vi "Computer.vi"() -> ()   [LabVIEW 2012]
uses:
  <vilib>/Utility/inputDevices.llb/closeJoystick.vi
  <vilib>/Utility/inputDevices.llb/joystickAcquire.vi
panel:
  out "TX Data":T1
  in  "ESTOP":bool
  in  "Robot Port":u16=2055 min=1025 step=1
  in  "Robot Address":string="192.168.1.200"
  in  "stop":bool
  # "Computer Control"
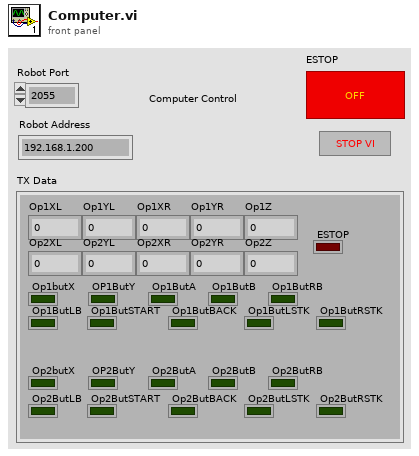
[diagram p1: front panel]
types:
  T1 = cluster{"Op2ButLSTK":bool, "Op2ButRSTK":bool, "Op1ButLSTK":bool, "Op1ButRSTK":bool, "Op1XL":i32, "Op1YL":i32, "Op1XR":i32, "Op1YR":i32, "Op1Z":i32, "Op2XL":i32, "Op2YL":i32, "Op2XR":i32, "Op2YR":i32, "Op2Z":i32, "ESTOP":bool, "Op1butX":bool, "OP1ButY":bool, "Op1ButA":bool, "Op1ButB":bool, "Op1ButRB":bool, "Op1ButLB":bool, "Op2butX":bool, "OP2ButY":bool, "Op2ButA":bool, "Op2ButB":bool, "Op2ButRB":bool, "Op2ButLB":bool, "Op2ButSTART":bool, "Op2ButBACK":bool, "Op1ButSTART":bool, "Op1ButBACK":bool}
  T2 = cluster{"X axis":i32, "Y axis":i32, "Z axis":i32, "X axis rotation":i32, "Y axis rotation":i32, "Z axis rotation":i32, "U axis":i32, "V axis":i32}
  T3 = cluster{"button 1":bool, "button 2":bool, "button 3":bool, "button 4":bool, "button 5":bool, "button 6":bool, "button 7":bool, "button 8":bool, "button 9":bool, "button 10":bool, "button 11":bool, "button 12":bool, "button 13":bool, "button 14":bool, "button 15":bool, "button 16":bool, "button 17":bool, "button 18":bool, "button 19":bool, "button 20":bool, "button 21":bool, "button 22":bool, "button 23":bool, "button 24":bool, "button 25":bool, "button 26":bool, "button 27":bool, "button 28":bool, "button 29":bool, "button 30":bool, "button 31":bool, "button 32":bool}
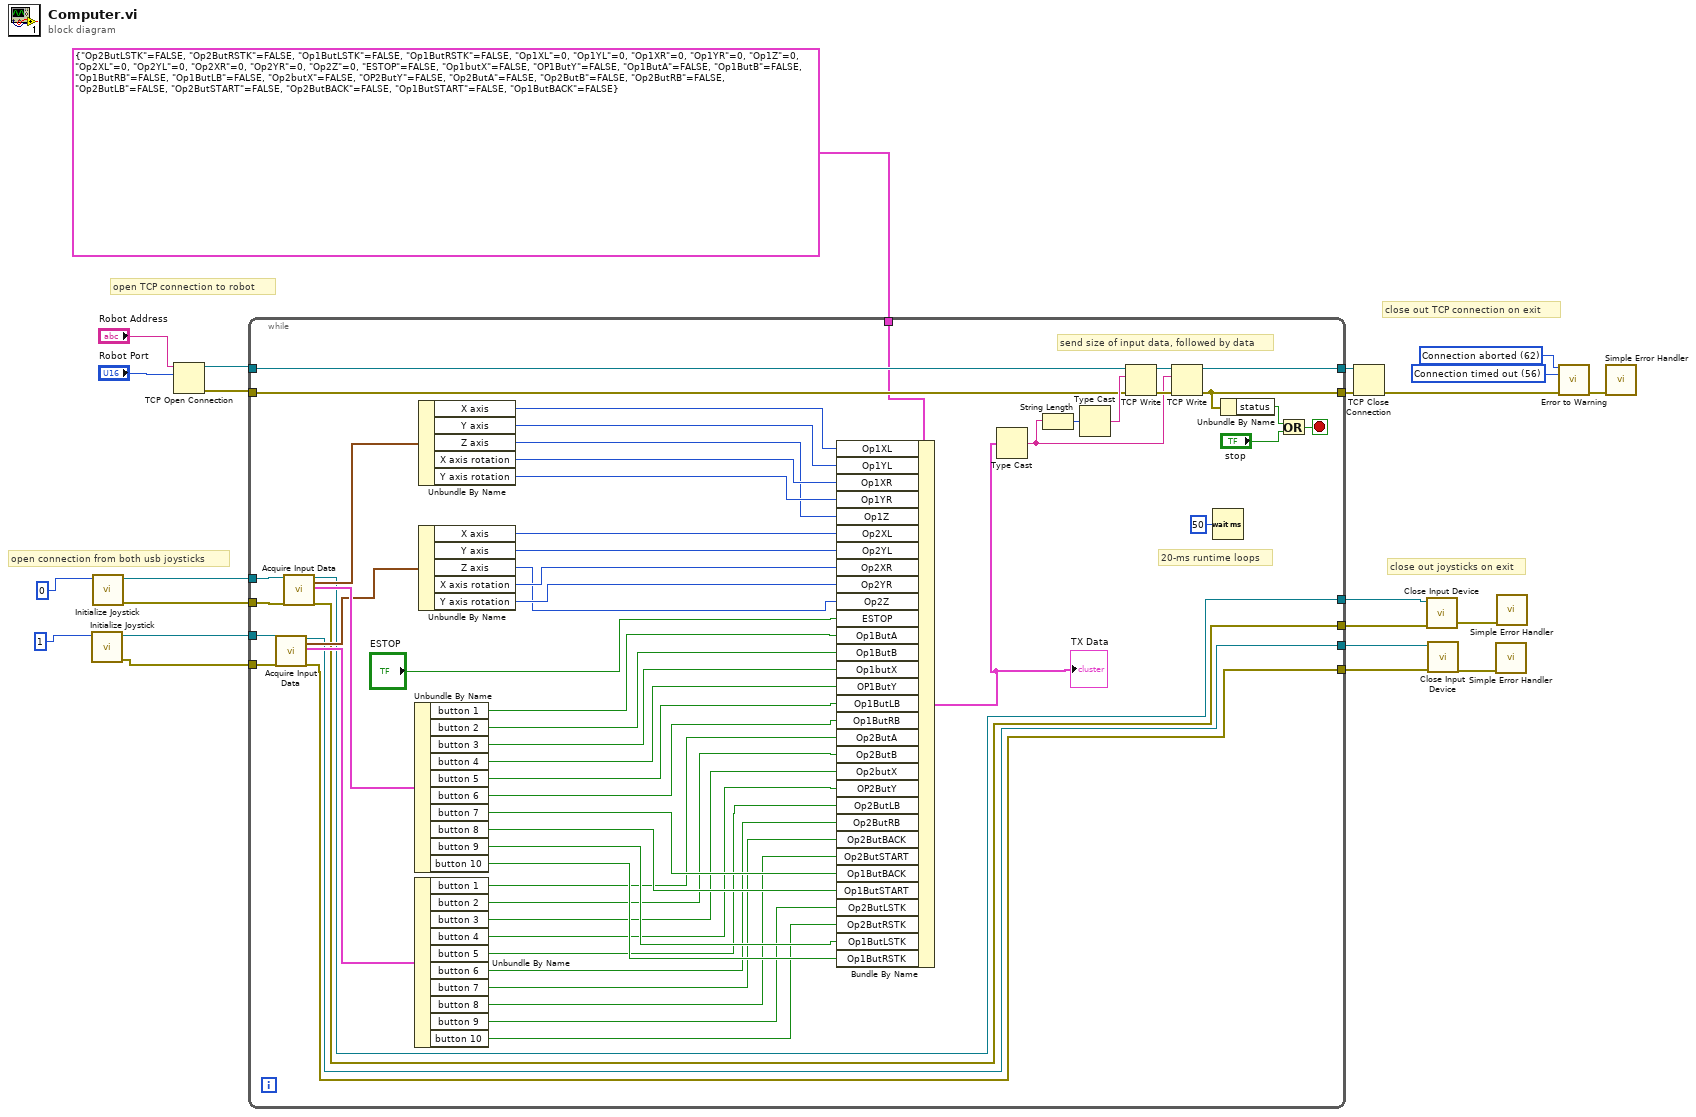
[diagram p0: block diagram]
diagram:
  w20 = 56 items=["No Error", "Argument Error", "Memory Full", "Out of Zone", "End of File", "File Already Open", "Generic File IO Error", "File Not Found", "File Permission Error", "Disk Full", "Duplicate Path", "Too Many Files Open", "Not Enabled", "Resource File Not Found", "Cannot Add Resource", "Resource Not Found", "Image Not Found", "Image Memory Error", "Pen Does Not Exist", "Config Bad Type", "Config Token Not Found", "Config Parse Error", "Config Memory Error", "Bad External Code Format", "Bad External Code Offset", "External Code Not Present", "Null Window", "Destroy Window Mixup", "Null Menu", "Print Aborted", "Bad Print Record", "Print Driver Error", "Windows Error During Print", "Memory Error During Print", "Print Dialog Error", "Generic Print Error", "Invalid Device Refnum", "Device Not Found", "Device Parameter Error", "Device Unit Error", "Can't Open Device", "Device Call Aborted", "Generic Error", "Cancelled By User", "Object ID Too Low", "Object ID Too High", "Object Not In Heap", "Unknown Heap", "Bad DefProc ID", "DefProc Not In Table", "Message Out Of Range", "Null Method", "Unknown Message", "Manager Call Not Supported", "Bad address", "Connection In progress", "Connection timed out", "Connection is already in progress", "Network attribute not supported", "Network error", "Address in use", "System out of memory", "Connection aborted", "Connection refused", "Connection is not connected", "Connection is already connected", "Connection closed", "Initialize error (interapplication manager)", "Bad occurrence", "Wait on unbound occurrence handler", "Occurrence queue overflow", "Bad path", "Semaphore not signaled", "Unrecognized type (interapplication manager)"] ("2nd Error to Convert")
  w21 = 62 items=["No Error", "Argument Error", "Memory Full", "Out of Zone", "End of File", "File Already Open", "Generic File IO Error", "File Not Found", "File Permission Error", "Disk Full", "Duplicate Path", "Too Many Files Open", "Not Enabled", "Resource File Not Found", "Cannot Add Resource", "Resource Not Found", "Image Not Found", "Image Memory Error", "Pen Does Not Exist", "Config Bad Type", "Config Token Not Found", "Config Parse Error", "Config Memory Error", "Bad External Code Format", "Bad External Code Offset", "External Code Not Present", "Null Window", "Destroy Window Mixup", "Null Menu", "Print Aborted", "Bad Print Record", "Print Driver Error", "Windows Error During Print", "Memory Error During Print", "Print Dialog Error", "Generic Print Error", "Invalid Device Refnum", "Device Not Found", "Device Parameter Error", "Device Unit Error", "Can't Open Device", "Device Call Aborted", "Generic Error", "Cancelled By User", "Object ID Too Low", "Object ID Too High", "Object Not In Heap", "Unknown Heap", "Bad DefProc ID", "DefProc Not In Table", "Message Out Of Range", "Null Method", "Unknown Message", "Manager Call Not Supported", "Bad address", "Connection In progress", "Connection timed out", "Connection is already in progress", "Network attribute not supported", "Network error", "Address in use", "System out of memory", "Connection aborted", "Connection refused", "Connection is not connected", "Connection is already connected", "Connection closed", "Initialize error (interapplication manager)", "Bad occurrence", "Wait on unbound occurrence handler", "Occurrence queue overflow", "Bad path", "Semaphore not signaled", "Unrecognized type (interapplication manager)"] ("1st Error to Convert")
  # "close out joysticks on exit"
  # "close out TCP connection on exit"
  # "open connection from both usb joysticks"
  # "open TCP connection to robot"
  n1 = call <vilib>:"Initialize Joystick.vi"("device index"=1) -> ("error out"=w8:errorcluster, "device ID"=w9:refnum<k1>)  [unwired: 9 in]
  n2 = call <vilib>:"Initialize Joystick.vi"("device index"=0) -> ("error out"=w12:errorcluster, "device ID"=w13:refnum<k1>)  [unwired: 9 in]
  n3 = TCP Open Connection(address="Robot Address", remote port or service name="Robot Port") -> (connection ID=w15:refnum<k5>, error out=w14:errorcluster)  [unwired: 3 in]
  n4 = while {
    tunnel: [w73] -> w18
    tunnel: [w81] -> w19
    tunnel: w15 -> [w80]
    tunnel: w14 -> [w70]
    tunnel: w13 -> [w68]
    tunnel: w12 -> [w67]
    tunnel: T1 {"Op2ButLSTK"=FALSE, "Op2ButRSTK"=FALSE, "Op1ButLSTK"=FALSE, "Op1ButRSTK"=FALSE, "Op1XL"=0, "Op1YL"=0, "Op1XR"=0, "Op1YR"=0, "Op1Z"=0, "Op2XL"=0, "Op2YL"=0, "Op2XR"=0, "Op2YR"=0, "Op2Z"=0, "ESTOP"=FALSE, "Op1butX"=FALSE, "OP1ButY"=FALSE, "Op1ButA"=FALSE, "Op1ButB"=FALSE, "Op1ButRB"=FALSE, "Op1ButLB"=FALSE, "Op2butX"=FALSE, "OP2ButY"=FALSE, "Op2ButA"=FALSE, "Op2ButB"=FALSE, "Op2ButRB"=FALSE, "Op2ButLB"=FALSE, "Op2ButSTART"=FALSE, "Op2ButBACK"=FALSE, "Op1ButSTART"=FALSE, "Op1ButBACK"=FALSE} -> [w66]
    tunnel: w9 -> [w29]
    tunnel: w8 -> [w28]
    tunnel: [w27] -> w6
    tunnel: [w26] -> w5
    tunnel: [w25] -> w4
    tunnel: [w24] -> w3
    stop <- w72 stop-if-true
    # "send size of input data, followed by data"
    # "20-ms runtime loops"
    n5 = call-poly <vilib>:"Acquire Input Data.vi"("device ID"=w29, "error in (no error)"=w28) -> ("device ID"=w26:refnum<k1>, "axis info"=w30:T2, "button info"=w31:T3, "error out"=w24:errorcluster)  [unwired: 13 in, 1 out]
    n6 = call-poly <vilib>:"Acquire Input Data.vi"("device ID"=w68, "error in (no error)"=w67) -> ("device ID"=w27:refnum<k1>, "axis info"=w49:T2, "button info"=w48:T3, "error out"=w25:errorcluster)  [unwired: 13 in, 1 out]
    n7 = Unbundle By Name(w48) -> ("button 1"=w59:bool, "button 2"=w58:bool, "button 3"=w57:bool, "button 4"=w56:bool, "button 5"=w55:bool, "button 6"=w54:bool, "button 7"=w53:bool, "button 8"=w52:bool, "button 9"=w51:bool, "button 10"=w50:bool)
    n8 = Unbundle By Name(w31) -> ("button 1"=w43:bool, "button 2"=w42:bool, "button 3"=w41:bool, "button 4"=w40:bool, "button 5"=w39:bool, "button 6"=w38:bool, "button 7"=w37:bool, "button 8"=w36:bool, "button 9"=w35:bool, "button 10"=w34:bool)
    n9 = Unbundle By Name(w49) -> ("X axis"=w63:i32, "Y axis"=w62:i32, "Z axis"=w33:i32, "X axis rotation"=w61:i32, "Y axis rotation"=w60:i32)
    n10 = Unbundle By Name(w30) -> ("X axis"=w47:i32, "Y axis"=w46:i32, "Z axis"=w32:i32, "X axis rotation"=w45:i32, "Y axis rotation"=w44:i32)
    n11 = Bundle By Name(cluster=w66, "Op1XL"=w63, "Op1YL"=w62, "Op1XR"=w61, "Op1YR"=w60, "Op1Z"=w33, "Op2XL"=w47, "Op2YL"=w46, "Op2XR"=w45, "Op2YR"=w44, "Op2Z"=w32, "ESTOP"="ESTOP", "Op1ButA"=w59, "Op1ButB"=w58, "Op1butX"=w57, "OP1ButY"=w56, "Op1ButLB"=w55, "Op1ButRB"=w54, "Op2ButA"=w43, "Op2ButB"=w42, "Op2butX"=w41, "OP2ButY"=w40, "Op2ButLB"=w39, "Op2ButRB"=w38, "Op2ButBACK"=w37, "Op2ButSTART"=w36, "Op1ButBACK"=w53, "Op1ButSTART"=w52, "Op2ButLSTK"=w35, "Op2ButRSTK"=w34, "Op1ButLSTK"=w51, "Op1ButRSTK"=w50) -> (w65:T1)
    "TX Data" <- w65
    n12 = Type Cast(x=w65) -> (*(type *) &x=w75:string)  [unwired: 1 in]
    n13 = String Length(string=w75) -> (length=w77:i32)
    n14 = Type Cast(x=w77) -> (*(type *) &x=w76:string)  [unwired: 1 in]
    n15 = TCP Write(connection ID=w80, data in=w76, error in (no error)=w70) -> (connection ID out=w79:refnum<k5>, error out=w78:errorcluster)  [unwired: 1 in, 1 out]
    n16 = TCP Write(connection ID=w79, data in=w75, error in (no error)=w78) -> (connection ID out=w81:refnum<k5>, error out=w73:errorcluster)  [unwired: 1 in, 1 out]
    n17 = Wait (ms)(milliseconds to wait=u32 50) -> ()  [unwired: 1 out]
    n18 = Unbundle By Name(w73) -> ("status"=w71:bool)
    n19 = Or(x=w71, y="stop") -> (x .or. y?=w72:bool)
  }
  n20 = TCP Close Connection(connection ID=w19, error in (no error)=w18) -> (error out=w23:errorcluster)  [unwired: 1 in, 1 out]
  n21 = call-poly <vilib>:"Close Input Device.vi"("error in (no error)"=w4, "device ID"=w6) -> ("error out"=w2:errorcluster)  [unwired: 8 in]
  n22 = call-poly <vilib>:"Close Input Device.vi"("error in (no error)"=w3, "device ID"=w5) -> ("error out"=w1:errorcluster)  [unwired: 8 in]
  n23 = call <vilib>:"Simple Error Handler.vi"("error in (no error)"=w1) -> ()  [unwired: 4 in, 5 out]
  n24 = call <vilib>:"Simple Error Handler.vi"("error in (no error)"=w2) -> ()  [unwired: 4 in, 5 out]
  n25 = call <vilib>:"Error to Warning.vi"("1st Error to Convert"=w21, "2nd Error to Convert"=w20, "error in"=w23) -> ("warning out"=w22:errorcluster)  [unwired: 12 in]
  n26 = call <vilib>:"Simple Error Handler.vi"("error in (no error)"=w22) -> ()  [unwired: 4 in, 5 out]
